vi "Load Config.vi"(6 "Constants":refnum<class "Sequence Constants.lvclass">, 8 "error in (no error)":refnum<class "MultiErrors.lvclass">, 10 "Config Element":refnum<class "Config Element.lvclass">, 11 "Inc Var Command Config in":refnum<class "Inc Var Command Config.lvclass">) -> (0 "error out":refnum<class "MultiErrors.lvclass">, 3 "Inc Var Command Config out":refnum<class "Inc Var Command Config.lvclass">)   [LabVIEW 2020, in "VolatusSeqConfig.lvlib" / "Inc Var Command Config.lvclass"]
uses:
  Inc Var Command Config.lvclass
  VolatusErrorUtilities/MultiErrors/MultiErrors.lvclass
  lv-cdm/CDM-Config/Config Element/Config Element.lvclass
  Sequence Constants/Sequence Constants.lvclass
  Inc Var Command Config.lvclass/Inc Var Command Config.ctl
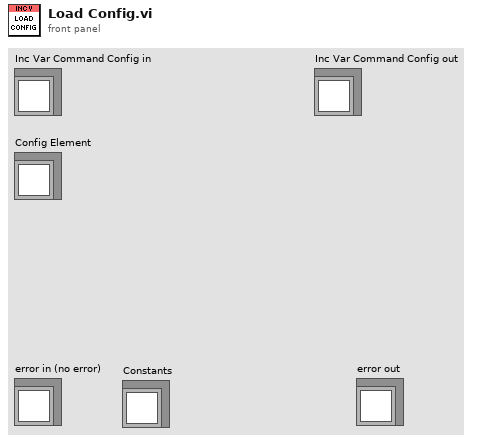
[diagram p1: front panel]
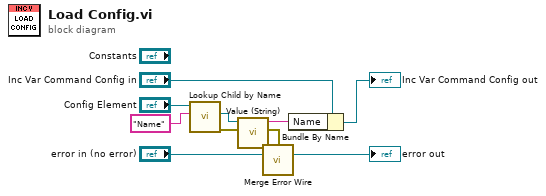
[diagram p0: block diagram]
diagram:
  n1 = call "Lookup Child by Name.vi"("Name"="Name", "Config Element in"="Config Element") -> ("error out"=w7:errorcluster, "Child"=w6:refnum<class "Config Element.lvclass">)  [unwired: 6 in, 2 out]
  n2 = call "Value (String).vi"("error in (no error)"=w7, "Config Element in"=w6) -> ("error out"=w1:errorcluster, "String Value"=w4:string)  [unwired: 8 in]
  n3 = call "Merge Error Wire.vi"("error in (no error)"=w1, "MultiErrors in"="error in (no error)") -> ("MultiErrors out"=→"error out":refnum<class "MultiErrors.lvclass">)  [unwired: 13 in]
  n4 = Bundle By Name(cluster="Inc Var Command Config in", "Name"=w4) -> (→"Inc Var Command Config out":refnum<class "Inc Var Command Config.lvclass">)
